vi "Execute.vi"(8 "error in (no error)":errorcluster, 10 "System In":refnum<class "abs_System.lvclass">, 11 "Node in":refnum<class "Not.lvclass">) -> (0 "error out":errorcluster, 1 "Status":T1, 2 "System Out":refnum<class "abs_System.lvclass">, 3 "Node out":refnum<class "Not.lvclass">)   [LabVIEW 2021, in "BT.lvlib" / "Not.lvclass"]
uses:
  Not.lvclass
  abs_Node/Status.ctl
  abs_System/abs_System.lvclass
  abs_Decorator/abs_Decorator.lvclass
  abs_Node/abs_Node.lvclass
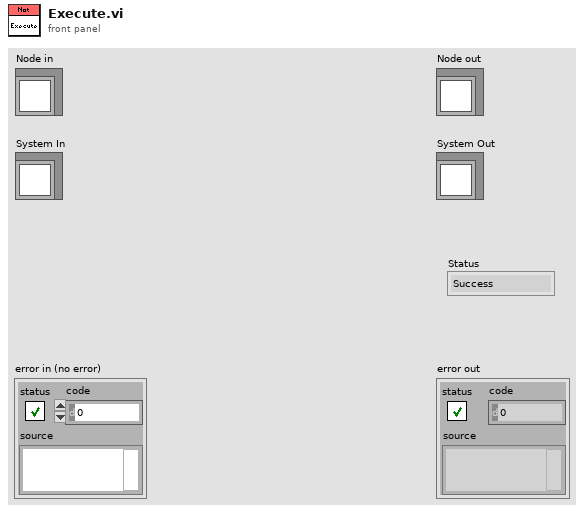
[diagram p1: front panel]
types:
  T1 = typedef "BT.lvlib/abs_Node.lvclass/Status.ctl" = enum16{"Success", "Failure", "Running"}
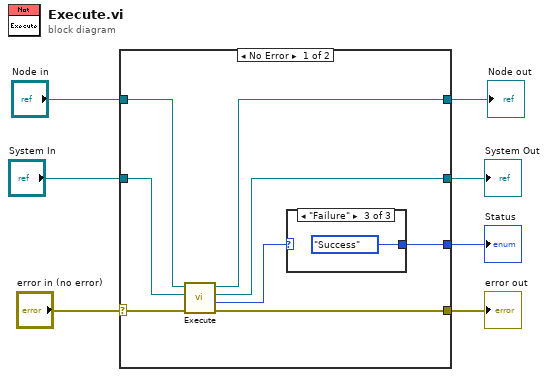
[diagram p0: block diagram]
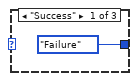
[diagram p2: hidden frame]
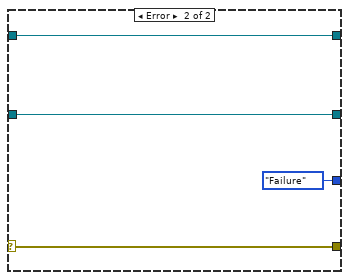
[diagram p4: hidden frame]
diagram:
  n1 = case shown="No Error" "error in (no error)" {
    selector: "error in (no error)" -> [w14 w20]
    tunnel: [w15 w21] -> w7
    tunnel: "System In" -> [w13 w21]
    tunnel: "Node in" -> [w12 w22]
    tunnel: [w11 w20] -> w3
    tunnel: [w10 w22] -> w2
    tunnel: [w8 Status."Failure" ("Status")] -> w1
    frame No Error {
      n2 = call-parent "Execute.vi"("error in (no error)"=w14, "System In"=w13, "Node in"=w12) -> ("error out"=w11:errorcluster, "Status"=w9:T1, "System Out"=w15:refnum<class "abs_System.lvclass">, "Node out"=w10:refnum<class "Not.lvclass">)  [unwired: 5 in]
      n3 = case shown="\"Failure\"" w9 {
        selector: w9 -> [_ w17 _]
        tunnel: [Status."Failure" ("Status") w17 Status."Success" ("Status")] -> w8
        frame "Success" {
        }
        frame "Running" {
        }
        frame "Failure" {
        }
      }
    }
    frame Error {
    }
  }
  "error out" <- w3
  "Node out" <- w2
  "Status" <- w1
  "System Out" <- w7
